vi "SwitchLane.vi"(10 "lane0":i32, 11 "Desired Lane":string) -> (2 "lane":i32, 3 "Switch":cluster{"SwitchRight":bool, "SwitchLeft":bool})   [LabVIEW 2013]
uses:
  <vilib>/imath/engines/lvmath2/RunTimeEngine/ErrorHandling/NIMS_Finalize Error.vi
  <vilib>/imath/engines/lvmath2/RunTimeEngine/Managers/WorkSpace/UID Generator.vi
  <vilib>/imath/engines/lvmath2/RunTimeEngine/VariableToken/NIMS_VariableToken_CondDefined.vi
  <instcachedir>/0/NIMS_VariableToken_CondDefined_9DC5CEC47F8146B087FA2781C705B229.lvgen/NIMS_VariableToken_CondDefined_9DC5CEC47F8146B087FA2781C705B229_003.vi
  <vilib>/imath/engines/lvmath/Functions/Error Handling/MergeErrorsWrapper.vi
  <vilib>/imath/engines/lvmath2/RunTimeEngine/Managers/SymbolTable/Clear UID.vi
  <vilib>/imath/engines/lvmath2/RunTimeEngine/NodeEndStatement/NIMS_NodeEndStatement_Output.vi
  <instcachedir>/0/NIMS_NodeEndStatement_Output_53EC0D466D134D7ABD903AC30B43404B.lvgen/NIMS_NodeEndStatement_Output_53EC0D466D134D7ABD903AC30B43404B_011.vi
  <instcachedir>/0/NIMS_NodeEndStatement_Output_53EC0D466D134D7ABD903AC30B43404B.lvgen/NIMS_NodeEndStatement_Output_53EC0D466D134D7ABD903AC30B43404B_010.vi
  <vilib>/imath/engines/lvmath2/RunTimeEngine/RunTimeType/NIMS_RunTimeType_From StrictType (excl LVString).vi
  <instcachedir>/0/NIMS_RunTimeType_From StrictType (excl LVString)_4DEE718D6EB74582AA20236969C084FC.lvgen/NIMS_RunTimeType_From StrictType (excl LVString)_4DEE718D6EB74582AA20236969C084FC_000.vi
  <vilib>/imath/engines/lvmath2/RunTimeEngine/LocalVariableDefStatement/MC_LocalVariableDefStatement_Display.vi
  <vilib>/imathl/engines/lvmath/Functions/Error Handling/Create Error.vi
  <vilib>/imath/engines/lvmath2/RunTimeEngine/Managers/SymbolTable/NIMS_WorkSpace.lvlib
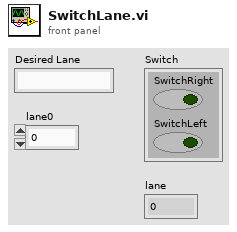
[diagram p1: front panel]
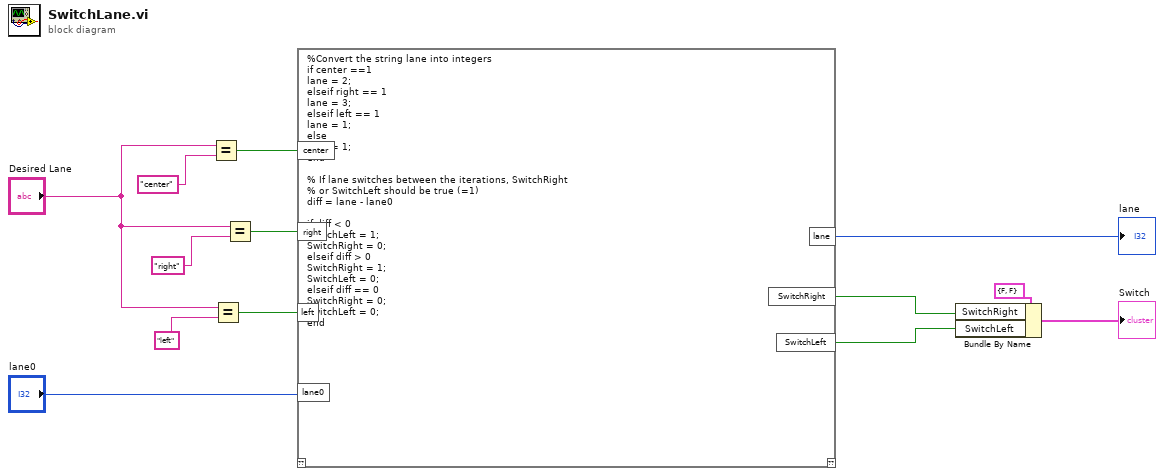
[diagram p0: block diagram]
diagram:
  n1 = Equal?(x="Desired Lane", y="center") -> (x = y?=w8:bool)
  n2 = Equal?(x="Desired Lane", y="left") -> (x = y?=w9:bool)
  n3 = Equal?(x="Desired Lane", y="right") -> (x = y?=w10:bool)
  n4 = mathscript code="%Convert the string lane into integers\nif center ==1\nlane = 2;\nelseif right == 1\nlane = 3;\nelseif left == 1\nlane = 1;\nelse\nlane = 1;\nend\n\n% If lane switches between the iterations, SwitchRight \n% or SwitchLeft should be true (=1)\ndiff = lane - lane0\n\nif diff < 0\nSwitchLeft = 1;\nSwitchRight = 0;\nelseif diff > 0 \nSwitchRight = 1;\nSwitchLeft = 0;\nelseif diff == 0\nSwitchRight = 0;\nSwitchLeft = 0;\nend"("center"=w8, "right"=w10, "left"=w9, "lane0"="lane0") -> ("lane"=→"lane":i32, "SwitchRight"=w2:bool, "SwitchLeft"=w1:bool)  [unwired: 1 in, 1 out]
  n5 = Bundle By Name(cluster=cluster{"SwitchRight":bool, "SwitchLeft":bool} {"SwitchRight"=FALSE, "SwitchLeft"=FALSE} ("Switch"), "SwitchRight"=w2, "SwitchLeft"=w1) -> (→"Switch":cluster{"SwitchRight":bool, "SwitchLeft":bool})
